vi "Read Status.vi"(8 "error in (no error)":errorcluster, 11 "Status Data in":refnum<class "Status Data.lvclass">) -> (0 "error out":errorcluster, 2 "Status":string, 3 "Status Data out":refnum<class "Status Data.lvclass">)   [LabVIEW 2020, in "Status Data.lvclass"]
uses:
  Status Data.lvclass
  Status Data.lvclass/Status Data.ctl
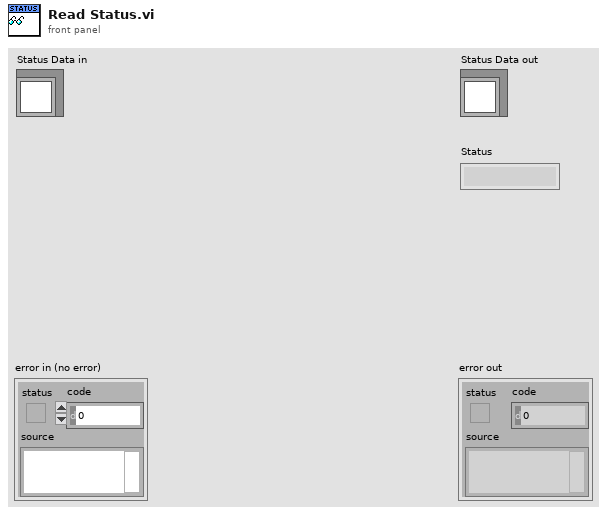
[diagram p1: front panel]
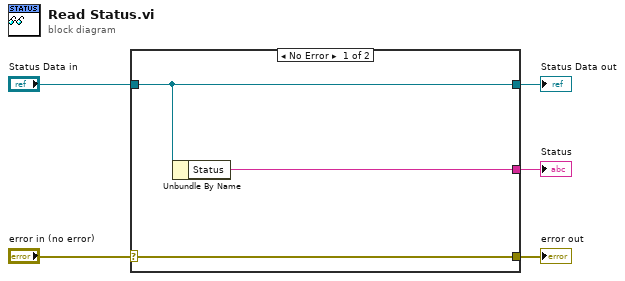
[diagram p0: block diagram]
diagram:
  n1 = case shown="No Error" "error in (no error)" {
    selector: "error in (no error)" -> [w8 w9]
    tunnel: [w8 w9] -> w4
    tunnel: [w7 w10] -> w2
    tunnel: "Status Data in" -> [w7 w10]
    tunnel: [w6 _] -> w1
    frame No Error {
      n2 = Unbundle By Name(w7) -> ("Status"=w6:string)
    }
    frame Error {
    }
  }
  "error out" <- w4
  "Status Data out" <- w2
  "Status" <- w1
